vi "Bradford Transformation.vi"(1 "XYZs":dbl[](array[numeric]), 2 "Illuminants":T1) -> (0 "XYZd":dbl[](array[numeric]) format="%.2f")   [LabVIEW 2013]
uses:
  <vilib>/Analysis/baseanly.llb/A x Vector.vi
  <vilib>/Analysis/baseanly.llb/Real A x B.vi
  <vilib>/Analysis/baseanly.llb/Real Inverse Matrix.vi
  <vilib>/Analysis/7linalg.llb/Create Special Real Matrix.vi
  <vilib>/Analysis/NI_AALBase.lvlib
  <vilib>/Analysis/NI_AALPro.lvlib
panel:
  out "WD":dbl[](array[numeric])
  out "WDe":bool
  out "WSe":bool
  out "WS":dbl[](array[numeric])
  out "Breadford Matrix":dbl[][](array[numeric])
  # "Chromatic Adaptation Evaluation"
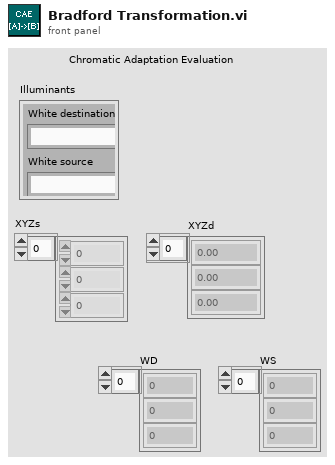
[diagram p1: front panel]
types:
  T1 = cluster{"White destination":string, "White source":string}
  T2 = typedef "NI_Matrix.lvlib/RealMatrix.ctl" = dbl[][]
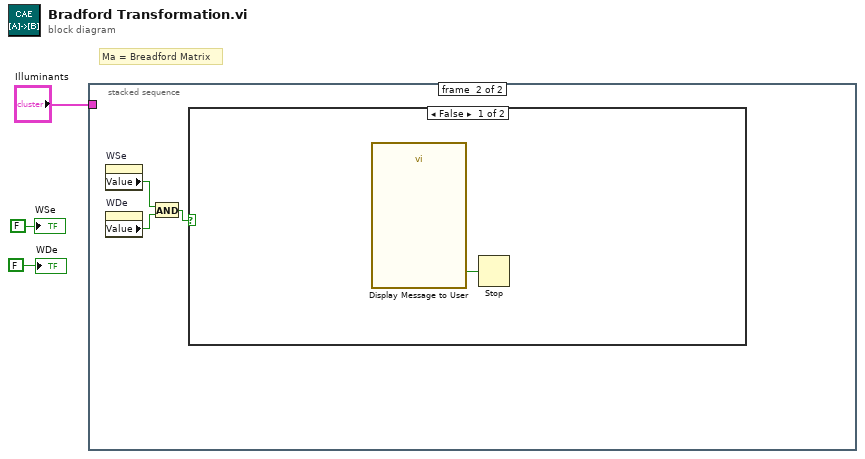
[diagram p0: block diagram]
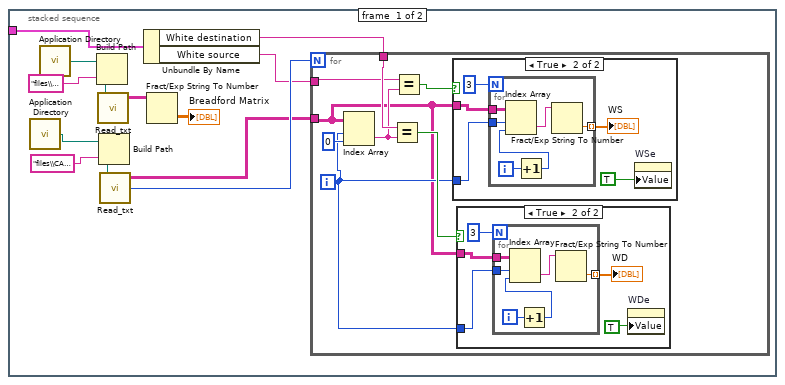
[diagram p2: hidden frame]
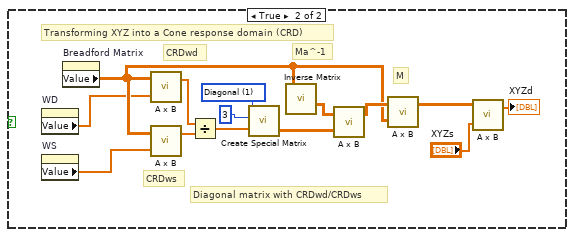
[diagram p5: hidden frame]
diagram:
  # "Ma = Breadford Matrix"
  n1 = stacked-sequence {
    tunnel: "Illuminants" -> [w8 _]
    frame #0 {
      n2 = call <vilib>:"Application Directory.vi"() -> ("Application Directory"=w4:path)
      n3 = call <vilib>:"Application Directory.vi"() -> ("Application Directory"=w5:path)
      n4 = Build Path(base path=w5, name or relative path="files\\Bradford.txt") -> (appended path=w15:path)
      n5 = call "Read_txt.vi"("file path (dialog if empty)"=w15) -> ("Elements"=w14:string[][])  [unwired: 2 out]
      n6 = Build Path(base path=w4, name or relative path="files\\CAS.txt") -> (appended path=w11:path)
      n7 = call "Read_txt.vi"("file path (dialog if empty)"=w11) -> ("Elements"=w9:string[][], "Rows"=w10:i32)  [unwired: 1 out]
      n8 = Unbundle By Name(w8) -> ("White destination"=w7:string, "White source"=w6:string)
      n9 = Fract/Exp String To Number(string=w14) -> (number=→"Breadford Matrix":dbl[][])  [unwired: 3 in, 1 out]
      n10 = for {
        N: w10 -> [_]
        tunnel: w9 -> [w17]
        tunnel: w7 -> [w24]
        tunnel: w6 -> [w23]
        i -> [w18]
        n11 = Index Array(array=w17, index (row)=w18, index (col)=0 ("disabled index (col)")) -> (element=w22:string)
        n12 = Equal?(x=w24, y=w22) -> (x = y?=w19:bool)
        n13 = Equal?(x=w23, y=w22) -> (x = y?=w20:bool)
        n14 = case shown="True" w20 {
          tunnel: w17 -> [_ w39]
          tunnel: w18 -> [_ w38]
          frame False {
          }
          frame True {
            n15 = for {
              N: 3 -> [_]
              tunnel: w39 -> [w46]
              tunnel: w38 -> [w45]
              tunnel: [w43] -> w37 mode=indexing
              i -> [w42]
              n16 = Increment(x=w42) -> (x+1=w41:i32)
              n17 = Index Array(array=w46, index (row)=w45, index (col)=w41) -> (element=w44:string)
              n18 = Fract/Exp String To Number(string=w44) -> (number=w43:dbl)  [unwired: 3 in, 1 out]
            }
            "WS" <- w37
            n19 = property on="WSe" class="Bool (strict)"("Value"=TRUE) -> ()  [unwired: 2 in, 2 out]
          }
        }
        n20 = case shown="True" w19 {
          tunnel: w17 -> [_ w28]
          tunnel: w18 -> [_ w27]
          frame False {
          }
          frame True {
            n21 = for {
              N: 3 -> [_]
              tunnel: w28 -> [w35]
              tunnel: w27 -> [w34]
              tunnel: [w32] -> w26 mode=indexing
              i -> [w30]
              n22 = Increment(x=w30) -> (x+1=w31:i32)
              n23 = Index Array(array=w35, index (row)=w34, index (col)=w31) -> (element=w33:string)
              n24 = Fract/Exp String To Number(string=w33) -> (number=w32:dbl)  [unwired: 3 in, 1 out]
            }
            "WD" <- w26
            n25 = property on="WDe" class="Bool (strict)"("Value"=TRUE) -> ()  [unwired: 2 in, 2 out]
          }
        }
      }
    }
    frame #1 {
      n26 = property on="WSe" class="Bool (strict)"() -> ("Value"=w48:bool)  [unwired: 2 in, 2 out]
      n27 = property on="WDe" class="Bool (strict)"() -> ("Value"=w47:bool)  [unwired: 2 in, 2 out]
      n28 = And(x=w48, y=w47) -> (x .and. y?=w49:bool)
      n29 = case shown="False" w49 {
        frame False {
          n30 = call "Display Message to User"() -> ("OK"=w50:bool)  [unwired: 10 in, 1 out]
          n31 = Stop(stop? (T)=w50) -> ()
        }
        frame True {
          w61 = 1 items=["Identity", "Diagonal", "Toeplitz", "Vandermonde", "Companion", "Hankel", "Hadamard", "Wilkinson", "Hilbert", "Inverse Hilbert", "Rosser", "Pascal"] ("matrix type")
          # "M"
          # "Diagonal matrix with CRDwd/CRDws"
          # "CRDws"
          # "CRDwd"
          # "Ma^-1"
          # "Transforming XYZ into a Cone response domain (CRD)"
          n32 = property on="WD" class="Arr (strict)"() -> ("Value"=w52:dbl[])  [unwired: 2 in, 2 out]
          n33 = property on="WS" class="Arr (strict)"() -> ("Value"=w53:dbl[])  [unwired: 2 in, 2 out]
          n34 = property on="Breadford Matrix" class="Arr (strict)"() -> ("Value"=w58:dbl[][])  [unwired: 2 in, 2 out]
          n35 = call-poly <vilib>:"A x B.vi"("Vector"=w52, "A"=w58) -> ("A x Vector"=w64:dbl[])  [unwired: 1 out]
          n36 = call-poly <vilib>:"A x B.vi"("Vector"=w53, "A"=w58) -> ("A x Vector"=w63:dbl[])  [unwired: 1 out]
          n37 = Divide(x=w64, y=w63) -> (x/y=w56:dbl[])
          n38 = call-poly <vilib>:"Create Special Matrix.vi"("matrix type"=w61, "matrix size"=3, "Input Vector1"=w56) -> ("Special Matrix"=w60:T2)  [unwired: 2 in, 1 out]
          n39 = call-poly <vilib>:"Inverse Matrix.vi"("Input Matrix"=w58) -> ("Inverse Matrix"=w57:T2)  [unwired: 1 in, 1 out]
          n40 = call-poly <vilib>:"A x B.vi"("B"=w60, "A"=w57) -> ("A x B"=w59:T2)  [unwired: 1 out]
          n41 = call-poly <vilib>:"A x B.vi"("B"=w58, "A"=w59) -> ("A x B"=w55:T2)  [unwired: 1 out]
          n42 = call-poly <vilib>:"A x B.vi"("Vector"="XYZs", "A"=w55) -> ("A x Vector"=→"XYZd":dbl[])  [unwired: 1 out]
        }
      }
    }
  }
  "WSe" <- FALSE ("WSe")
  "WDe" <- FALSE ("WSe")
